vi "conv_LHe_level.vi"(11 "level_in":dbl) -> (3 "level_out":dbl)   [LabVIEW 2019]
panel:
  # "The conversion formula was taken from UVA elog 153."
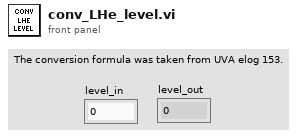
[diagram p1: front panel]
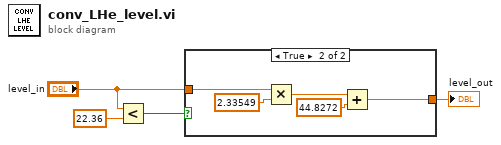
[diagram p0: block diagram]
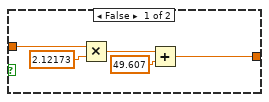
[diagram p2: hidden frame]
diagram:
  n1 = Less?(x="level_in", y=22.36) -> (x < y?=w3:bool)
  n2 = case shown="True" w3 {
    tunnel: "level_in" -> [w9 w11]
    tunnel: [w5 w10] -> w1
    frame False {
      n3 = Multiply(x=w9, y=2.12173) -> (x*y=w7:dbl)
      n4 = Add(x=w7, y=49.607) -> (x+y=w5:dbl)
    }
    frame True {
      n5 = Multiply(x=w11, y=2.33549) -> (x*y=w13:dbl)
      n6 = Add(x=w13, y=44.8272) -> (x+y=w10:dbl)
    }
  }
  "level_out" <- w1
